vi "综合实验一.vi"() -> ()   [LabVIEW 2018]
panel:
  out "当前湿度":dbl format="%#_4g"
  out "湿度量表":dbl(knob) scale=0.0..100.0 scale format="%#_4g"
  out "湿度趋势曲线图":dbl(graph)
  in  "湿度上限":i32=75
  in  "湿度下限":i32=40
  out "温度上限报警":bool
  out "温度下限报警":bool
  out "温度计":dbl(slide) scale=0.0..100.0 scale format="%#_4g"
  out "温度趋势曲线图":dbl(graph)
  out "当前温度":dbl format="%#_4g"
  in  "温度上限":i32=75
  in  "温度下限":i32=40
  out "湿度上限报警":bool
  out "湿度下限报警":bool
  out "系统指示灯":bool
  in  "退出系统":bool
  out "系统时间":timestamp
  out "数据显示":string
  in  "路径":path=path "F:/Labview实验/Labview实验/新建文本文档.txt"
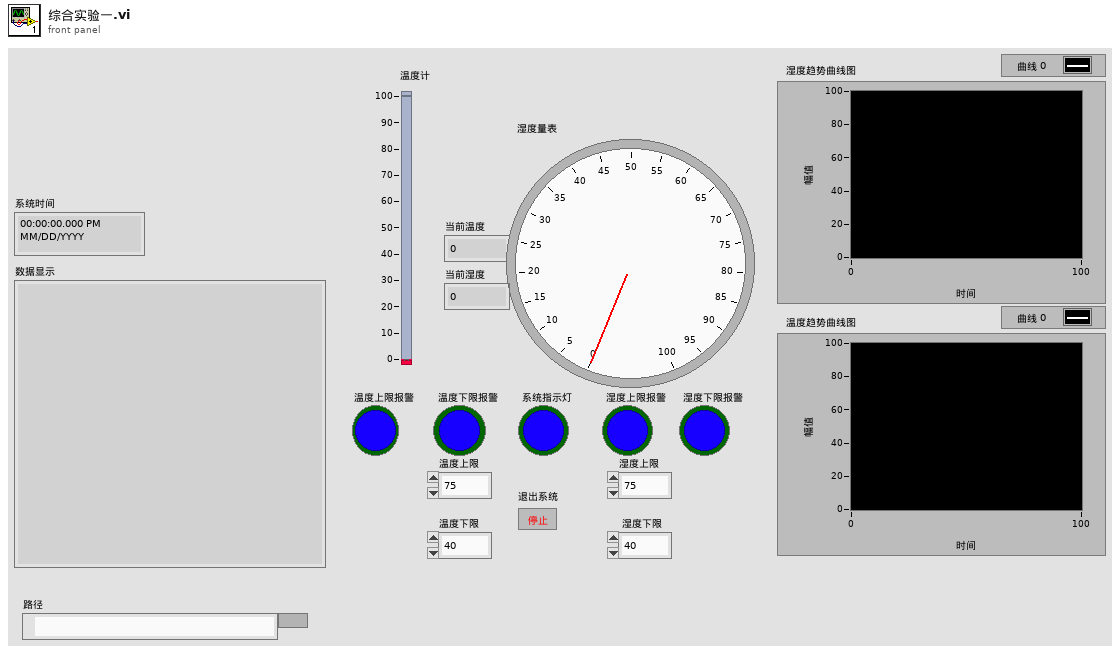
[diagram p1: front panel]
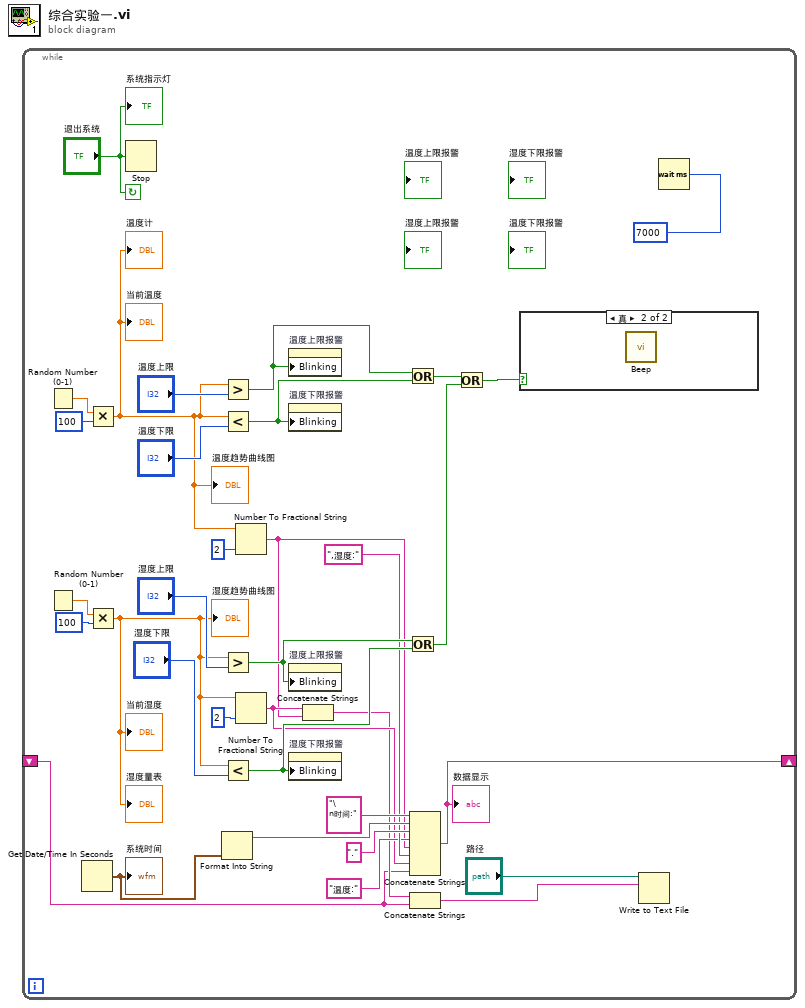
[diagram p0: block diagram]
diagram:
  n1 = while {
    shift-right: [w11] -> _
    shift-left: _ -> [w5]
    stop <- "退出系统" continue-if-true
    n2 = Random Number (0-1)() -> (number: 0 to 1=w18:dbl)
    n3 = Random Number (0-1)() -> (number: 0 to 1=w20:dbl)
    n4 = Get Date/Time In Seconds() -> (seconds since 1Jan1904=w23:timestamp)
    "系统时间" <- w23
    n5 = Multiply(x=w18, y=100) -> (x*y=w16:dbl)
    "温度计" <- w16
    "温度趋势曲线图" <- w16
    "当前温度" <- w16
    n6 = Multiply(x=w20, y=100) -> (x*y=w15:dbl)
    "当前湿度" <- w15
    "湿度量表" <- w15
    "湿度趋势曲线图" <- w15
    n7 = Stop(stop? (T)="退出系统") -> ()
    n8 = Format Into String(w23) -> (resulting string=w22:string)  [unwired: 3 in, 1 out]
    n9 = Greater?(x=w16, y="温度上限") -> (0:w3:bool)
    n10 = Less?(x=w16, y="温度下限") -> (x < y?=w30:bool)
    n11 = Greater?(x=w15, y="湿度上限") -> (0:w29:bool)
    n12 = Less?(x=w15, y="湿度下限") -> (x < y?=w28:bool)
    n13 = Number To Fractional String(number=w16, precision (6)=2) -> (F-format string=w9:string)  [unwired: 2 in]
    n14 = Number To Fractional String(number=w15, precision (6)=2) -> (F-format string=w10:string)  [unwired: 2 in]
    n15 = property on="温度上限报警" class="Bool (严格)"("Blinking"=w3) -> ()  [unwired: 2 in, 2 out]
    n16 = property on="温度下限报警" class="Bool (严格)"("Blinking"=w30) -> ()  [unwired: 2 in, 2 out]
    n17 = property on="湿度上限报警" class="Bool (严格)"("Blinking"=w29) -> ()  [unwired: 2 in, 2 out]
    n18 = property on="湿度下限报警" class="Bool (严格)"("Blinking"=w28) -> ()  [unwired: 2 in, 2 out]
    n19 = Concatenate Strings(w10, w9) -> (w8:string)
    n20 = Or(x=w3, y=w30) -> (x .or. y?=w27:bool)
    n21 = Or(x=w29, y=w28) -> (x .or. y?=w26:bool)
    n22 = Concatenate Strings("\n时间:", w22, ".", "温度:", w9, ",湿度:", w10, w5) -> (w11:string)
    "数据显示" <- w11
    n23 = Concatenate Strings(w8, w5) -> (w7:string)
    n24 = Or(x=w27, y=w26) -> (x .or. y?=w25:bool)
    n25 = case shown="真" w25 {
      frame False {
      }
      frame True {
        n26 = call <vilib>:"Beep.vi"() -> ()  [unwired: 12 in]
      }
    }
    n27 = Write to Text File(file (use dialog)="路径", text=w7) -> ()  [unwired: 2 in, 3 out]
    n28 = Wait (ms)(milliseconds to wait=7000) -> ()  [unwired: 1 out]
    "系统指示灯" <- "退出系统"
  }
